vi "Configure PowerSupply.vi"(0 "Address":string="8", 5 "error in (no error)":errorcluster) -> (6 "Address Out":string, 8 "error out":errorcluster)   [LabVIEW 2017]
panel:
  in  "Enable":bool=TRUE
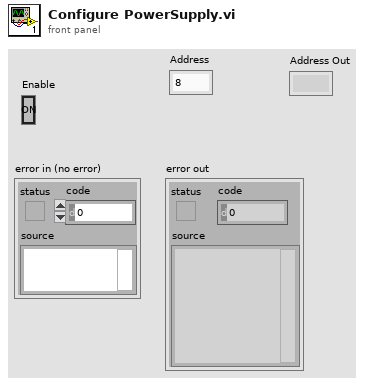
[diagram p1: front panel]
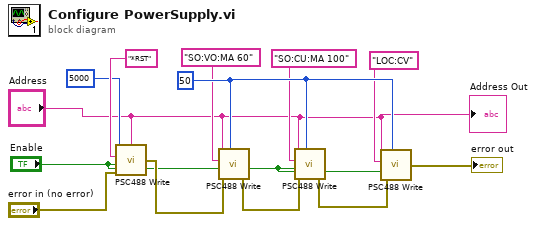
[diagram p0: block diagram]
diagram:
  w6 = u16 50 ("Delay")
  n1 = call "PSC488 Write.vi"("Address"="Address", "Command"="*RST", "Enable"="Enable", "error in (no error)"="error in (no error)", "Delay after write"=u16 5000 ("Delay")) -> ("error out"=w11:errorcluster)
  n2 = call "PSC488 Write.vi"("Address"="Address", "Command"="SO:VO:MA 60", "Enable"="Enable", "error in (no error)"=w11, "Delay after write"=w6) -> ("error out"=w10:errorcluster)
  n3 = call "PSC488 Write.vi"("Address"="Address", "Command"="SO:CU:MA 100", "Enable"="Enable", "error in (no error)"=w10, "Delay after write"=w6) -> ("error out"=w8:errorcluster)
  n4 = call "PSC488 Write.vi"("Address"="Address", "Command"="LOC:CV", "Enable"="Enable", "error in (no error)"=w8, "Delay after write"=w6) -> ("error out"=→"error out":errorcluster)
  "Address Out" <- "Address"
